vi "CALC_Mean_pixel_gauss_values.vi"(7 "Interp. steps":i32=100, 8 "error in (no error)":errorcluster, 9 "Sigma":dbl=1.0, 10 "Y":dbl, 11 "X":dbl) -> (0 "error out":errorcluster, 2 "Interp. step gaussian values":dbl[][](array[numeric]), 3 "Average interp. gaussian value":dbl)   [LabVIEW 2018, in "Tracker.lvlib"]
uses:
  Tracker.lvlib
  <vilib>/Analysis/baseanly.llb/Mean (DBL).vi
  <vilib>/express/express arith-compare/Formula/XNode/ExpressFormulaBlockNode.xnode
  <vilib>/Analysis/NI_AALBase.lvlib
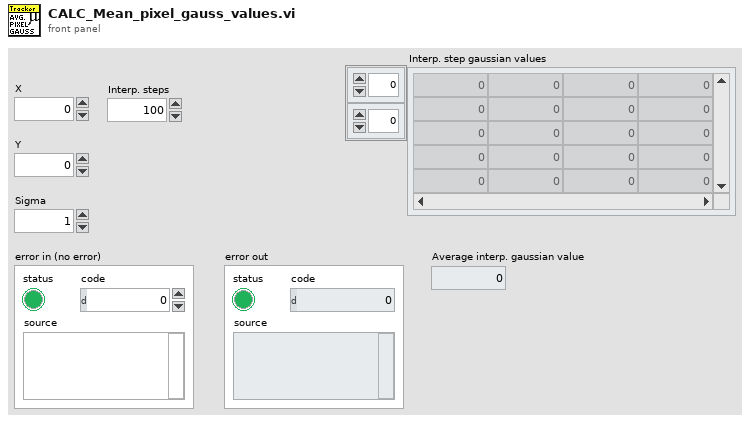
[diagram p1: front panel]
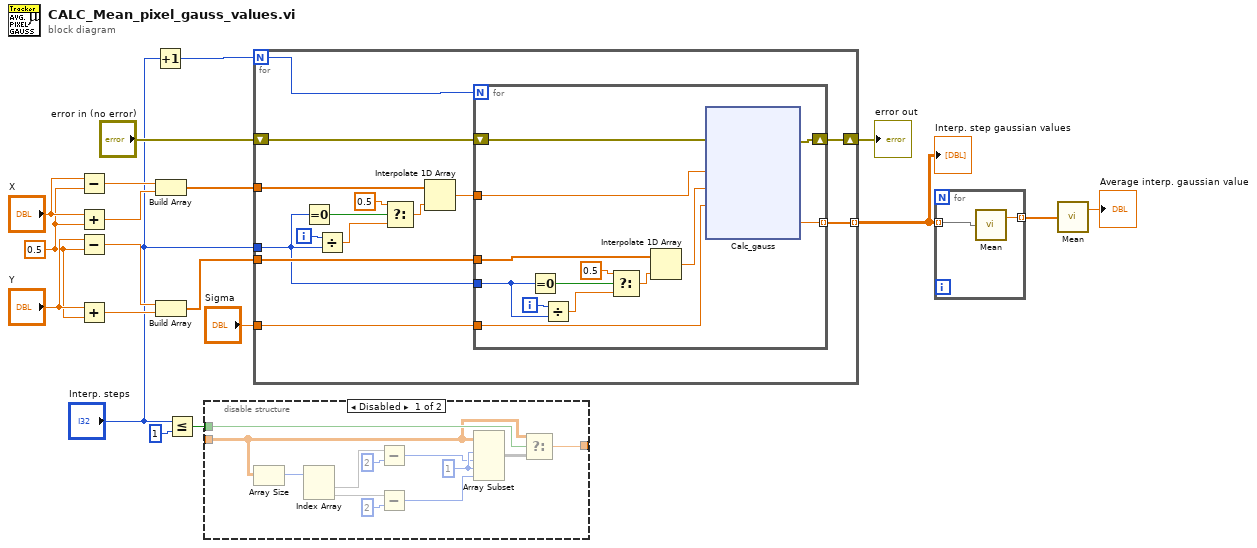
[diagram p0: block diagram]
diagram:
  w15 = 0.5
  n1 = Subtract(x="X", y=w15) -> (x-y=w14:dbl)
  n2 = Add(x="X", y=w15) -> (x+y=w13:dbl)
  n3 = Subtract(x="Y", y=w15) -> (x-y=w12:dbl)
  n4 = Add(x="Y", y=w15) -> (x+y=w11:dbl)
  n5 = Increment(x="Interp. steps") -> (x+1=w8:i32)
  n6 = Build Array(w14, w13) -> (w10:dbl[])
  n7 = Build Array(w12, w11) -> (w9:dbl[])
  n8 = Less Or Equal?(x="Interp. steps", y=1) -> (x <= y?=w4:bool)
  n9 = disable-structure shown="Disabled" {
    disable-tunnel: w4 -> [w23 _]
    disable-tunnel: [w21 _] -> _
    disable-tunnel: _ -> [w20 _]
    frame Disabled {
      w30 = 1 ("index")
      n10 = Array Size(array=w20) -> (size(s)=w31:i32)
      n11 = Index Array(array=w31) -> (element #1=w29, element #2=w25)  [unwired: 2 in]
      n12 = Subtract(x=w29, y=2 ("index")) -> (x-y=w27:i32)
      n13 = Subtract(x=w25, y=2 ("index")) -> (x-y=w24:i32)
      n14 = Array Subset(array=w20, index (row)=w30, length (row)=w27, index (col)=w30, length (col)=w24) -> (w22:void[][])
      n15 = Select(t=w20, s=w23, f=w22) -> (s? t:f=w21:dbl)
    }
    frame Enabled {
    }
  }
  n16 = for {
    N: w8 -> [w43]
    shift-right: [w45] -> w19
    shift-left: "error in (no error)" -> [w44]
    tunnel: w10 -> [w42]
    tunnel: w9 -> [w35]
    tunnel: "Interp. steps" -> [w34]
    tunnel: [w32] -> w1 mode=indexing
    tunnel: "Sigma" -> [w33]
    i -> [w41]
    n17 = Equal To 0?(x=w34) -> (x = 0?=w37:bool)
    n18 = Divide(x=w41, y=w34) -> (x/y=w38:dbl)
    n19 = Select(t=0.5, s=w37, f=w38) -> (s? t:f=w39:dbl)
    n20 = Interpolate 1D Array(1:w39, 2:w42) -> (0:w40:dbl)
    n21 = for {
      N: w43 -> [_]
      shift-right: [w58] -> w45
      shift-left: w44 -> [w57]
      tunnel: w40 -> [w56]
      tunnel: w35 -> [w51]
      tunnel: w34 -> [w49]
      tunnel: [w48] -> w32 mode=indexing
      tunnel: w33 -> [w46]
      i -> [w50]
      n22 = Equal To 0?(x=w49) -> (x = 0?=w54:bool)
      n23 = Divide(x=w50, y=w49) -> (x/y=w53:dbl)
      n24 = Select(t=0.5, s=w54, f=w53) -> (s? t:f=w52:dbl)
      n25 = Interpolate 1D Array(1:w52, 2:w51) -> (0:w47:dbl)
      n26 = xnode ("Calc_gauss")("X"=w56, "Y"=w47, "sigma"=w46, "error in (no error)"=w57) -> ("Result"=w48:dbl, "error out"=w58:errorcluster)
    }
  }
  "error out" <- w19
  "Interp. step gaussian values" <- w1
  n27 = for {
    tunnel: w1 -> [w72] mode=indexing
    tunnel: [w71] -> w6 mode=indexing
    n28 = call-poly <vilib>:"Mean.vi"("X"=w72) -> ("mean"=w71:dbl)  [unwired: 1 out]
  }
  n29 = call-poly <vilib>:"Mean.vi"("X"=w6) -> ("mean"=→"Average interp. gaussian value":dbl)  [unwired: 1 out]
